vi "Allocate Complex Cluster.vi"(0 "Seconds\nper Frame":dbl=0.2, 1 "Actual Rx Parameters":T1) -> (2 "Rx IQ Sampling\nRate [s/sec]":dbl, 3 "Allocated Cluster":cluster{"t0":dbl, "dt":dbl, "Y":cdb[]}, 4 "Number of Samples":i32)   [LabVIEW 2010]
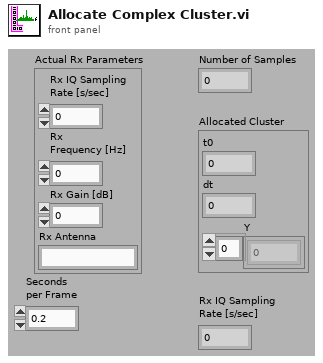
[diagram p1: front panel]
types:
  T1 = cluster{"Rx IQ Sampling\nRate [s/sec]":dbl, "Rx\nFrequency [Hz]":dbl, "Rx Gain [dB]":dbl, "Rx Antenna":string}
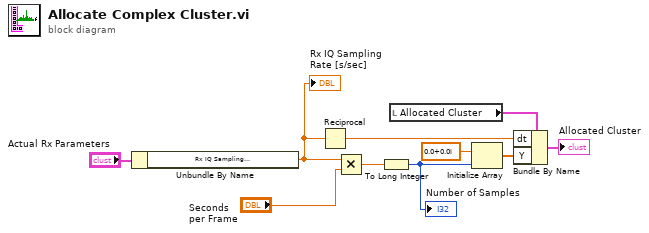
[diagram p0: block diagram]
diagram:
  n1 = Unbundle By Name("Actual Rx Parameters") -> ("Rx IQ Sampling\nRate [s/sec]"=w3:dbl)
  "Rx IQ Sampling\nRate [s/sec]" <- w3
  n2 = Reciprocal(x=w3) -> (1/x=w4:dbl)
  n3 = Multiply(x=w3, y="Seconds\nper Frame") -> (x*y=w8:dbl)
  n4 = To Long Integer(number=w8) -> (32bit integer=w9:i32)
  "Number of Samples" <- w9
  n5 = local read "Allocated Cluster"() -> (w5:cluster{"t0":dbl, "dt":dbl, "Y":cdb[]})
  n6 = Initialize Array(cdb 0.0+0.0i ("element"), w9) -> (w2:cdb[])
  n7 = Bundle By Name(cluster=w5, "dt"=w4, "Y"=w2) -> (→"Allocated Cluster":cluster{"t0":dbl, "dt":dbl, "Y":cdb[]})
